vi "ConvertGPS-MDFtoXY-MDF.vi"(0 "5.1.1 MDF GPS":T1) -> (1 "XY Graph":cluster{ext[], ext[]}(graph), 2 "5.1.1 MDF XY":T1, 3 "Array of GPS coors":ext[][](array[numeric]))   [LabVIEW 2010]
uses:
  4-High Neurons/MDFArray.ctl
  6-OCU Neurons/MDF Waypoint.ctl
  5.0-Global.vi
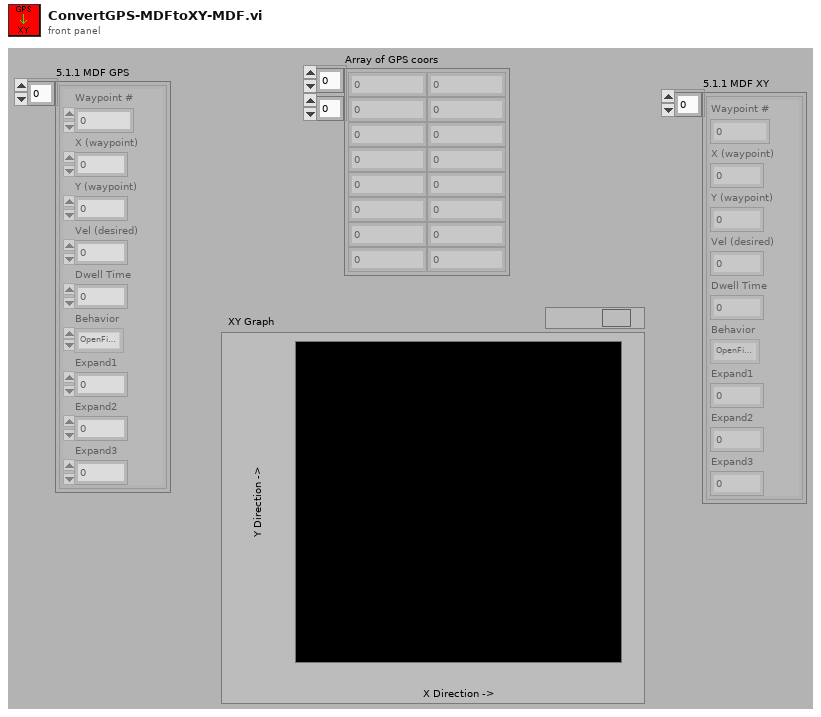
[diagram p1: front panel]
types:
  T1 = typedef "MDFArray.ctl" = T2[]
  T2 = typedef "MDF Waypoint.ctl" = cluster{"Waypoint #":dbl, "X (waypoint)":ext, "Y (waypoint)":ext, "Vel (desired)":dbl, "Dwell Time":dbl, "Behavior":enum16{"OpenFieldTransit", "WallFollow", "LaneFollow", "ManualMode"}, "Expand1":dbl, "Expand2":dbl, "Expand3":dbl}
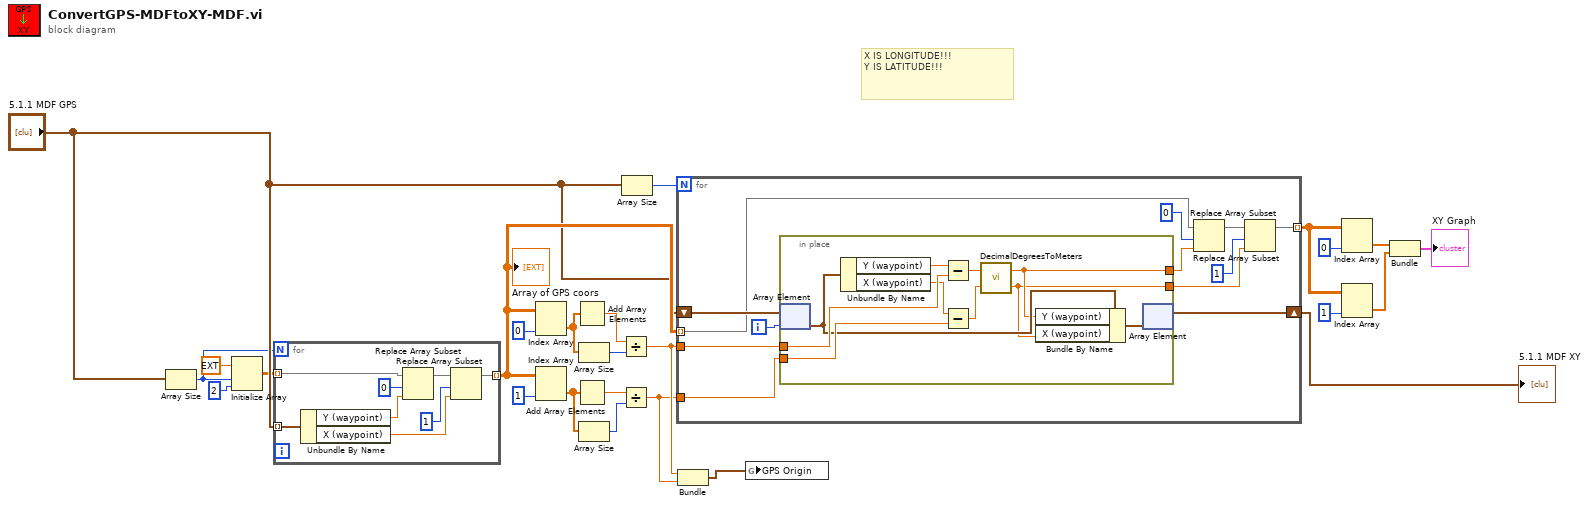
[diagram p0: block diagram]
diagram:
  # "X IS LONGITUDE!!!\nY IS LATITUDE!!!"
  n1 = Array Size(array="5.1.1 MDF GPS") -> (size(s)=w9:i32)
  n2 = Initialize Array(ext 0.0 ("element"), w9, 2 ("dimension size")) -> (w6:ext[][])
  n3 = for {
    N: w9 -> [_]
    tunnel: "5.1.1 MDF GPS" -> [w33] mode=indexing
    tunnel: w6 -> [w32] mode=indexing
    tunnel: [w30] -> w19 mode=indexing
    n4 = Unbundle By Name(w33) -> ("Y (waypoint)"=w29:ext, "X (waypoint)"=w26:ext)
    n5 = Replace Array Subset(array=w32, new element=w29, index=0 ("dimension size")) -> (w31:ext[])
    n6 = Replace Array Subset(array=w31, new element=w26, index=1 ("dimension size")) -> (w30:ext[])
  }
  "Array of GPS coors" <- w19
  n7 = Index Array(array=w19, index (col)=0 ("disabled index (col)")) -> (element=w12:ext[])  [unwired: 1 in]
  n8 = Index Array(array=w19, index (col)=1 ("disabled index (col)")) -> (element=w16:ext[])  [unwired: 1 in]
  n9 = Add Array Elements(numeric array=w12) -> (sum=w11:ext)
  n10 = Add Array Elements(numeric array=w16) -> (sum=w14:ext)
  n11 = Array Size(array=w12) -> (size(s)=w13:i32)
  n12 = Array Size(array=w16) -> (size(s)=w15:i32)
  n13 = Divide(x=w11, y=w13) -> (x/y=w3:ext)
  n14 = Divide(x=w14, y=w15) -> (x/y=w2:ext)
  n15 = Array Size(array="5.1.1 MDF GPS") -> (size(s)=w18:i32)
  n16 = for {
    N: w18 -> [_]
    shift-right: [w44] -> w10
    shift-left: "5.1.1 MDF GPS" -> [w45]
    tunnel: w3 -> [w43]
    tunnel: w2 -> [w42]
    tunnel: w19 -> [w40] mode=indexing
    tunnel: [w34] -> w20 mode=indexing
    i -> [w41]
    n17 = in-place {
      in-place-border: w43 -> [w54]
      in-place-border: w42 -> [w52]
      in-place-border: [w47] -> w36
      in-place-border: [w46] -> w35
      n18 = in-place-array #1(w45, w41) -> (w51:T2)
      n19 = Unbundle By Name(w51) -> ("Y (waypoint)"=w55:ext, "X (waypoint)"=w53:ext)
      n20 = Subtract(x=w55, y=w54) -> (x-y=w49:ext)
      n21 = Subtract(x=w53, y=w52) -> (x-y=w48:ext)
      n22 = call "DecimalDegreesToMeters.vi"("Longitude"=w48, "Latitude"=w49) -> ("X"=w46:dbl, "Y"=w47:dbl)
      n23 = Bundle By Name(cluster=w51, "Y (waypoint)"=w47, "X (waypoint)"=w46) -> (w50:T2)
      n24 = in-place-array #1(w50) -> (w44:T1)  [unwired: 1 out]
    }
    n25 = Replace Array Subset(array=w40, new element=w36, index=0) -> (w39:ext[])
    n26 = Replace Array Subset(array=w39, new element=w35, index=1) -> (w34:ext[])
  }
  "5.1.1 MDF XY" <- w10
  n27 = Bundle(w3, w2) -> (w1:cluster{ext, ext})  [unwired: 1 in]
  n28 = global write "5.0-Global.vi" "GPS Origin"(w1) -> ()
  n29 = Index Array(array=w20, index (col)=0 ("disabled index (col)")) -> (element=w21:ext[])  [unwired: 1 in]
  n30 = Index Array(array=w20, index (col)=1 ("disabled index (col)")) -> (element=w22:ext[])  [unwired: 1 in]
  n31 = Bundle(w21, w22) -> (→"XY Graph":cluster{ext[], ext[]})  [unwired: 1 in]
